vi "Process.vi"(8 "error in":errorcluster, 11 "SMO.Example":refnum<class "SMO.Example.lvclass">) -> (0 "error out":errorcluster, 3 "SMO.Example out":refnum<class "SMO.Example.lvclass">)   [LabVIEW 2013, in "SMO.Example.lvclass"]
doc: "---------------------------------------------------------------\nJKI State Machine Objects™\nhttp://jki.net/state-machine-objects/\nCopyright (C) 2005-2015, JKI <info@jki.net>\nALL RIGHTS RESERVED"
uses:
  SMO.Example.lvclass
  SMO/Typedefs/Parent Call--Enum.ctl
  SMO/SMO.lvclass
panel:
  # "For instructions on how to use the JKI State Machine Objects, examples and video tutorials, visit:\nhttp://jki.net/state-machine-objects/\n\nJKI State Machine Objects™\nhttp://jki.net/state-machine-objects/\nCopyright (C) 2005-2015, JKI <info@jki.net>\nALL RIGHTS RESERVED"
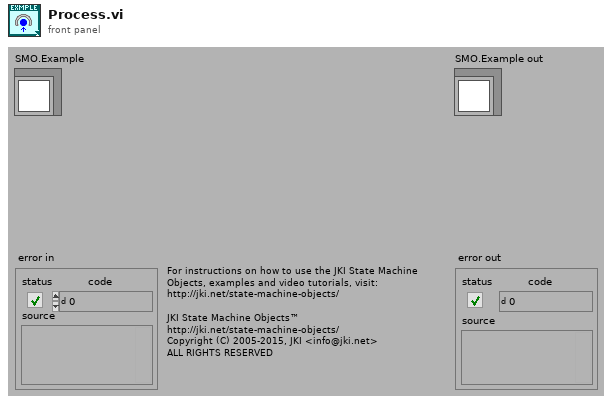
[diagram p1: front panel]
types:
  T1 = typedef "SMO.lvclass/Parent Call--Enum.ctl" = enum16{"Allows parent to run", "Does not request parent to run"}
  T2 = enum32{"invalid app kind", "Development System", "Run Time System", "Student Edition", "Embedded LabVIEW", "Evaluation", "Custom"}
  T3 = enum32{"Invalid", "Standard", "Closed", "Hidden", "Minimized", "Maximized"}
  T4 = enum32{"Bad", "Idle", "Run top level", "Running"}
  T5 = cluster{"Core":cluster{"Current VI Reference":refnum<vi>, "Close Panel on Exit?":bool, "error":errorcluster}, "Self Ref":refnum<class "SMO.Example.lvclass">, "Exec.State":enum32{"Bad", "Idle", "Run top level", "Running"}, "Your string data":string, "Pump State":bool, "Valve 1 State":bool, "Flow 1 Actual":dbl, "Flow 2 Actual":dbl, "Flow 1 Target":dbl, "Flow 2 Target":dbl}
  T6 = cluster{"Current VI Reference":refnum<vi>, "Close Panel on Exit?":bool, "error":errorcluster}
  T7 = typedef "SMO.lvclass/Protected Events.ctl" = cluster{"StopProcesses":refnum<user-event>, "AbortProcesses":refnum<user-event>}
  T8 = typedef "SMO.Example.lvclass/ProtectedEvents--Cluster.ctl" = cluster{"API_Template":refnum<user-event>, "PumpState":refnum<user-event>, "Valve State":refnum<user-event>}
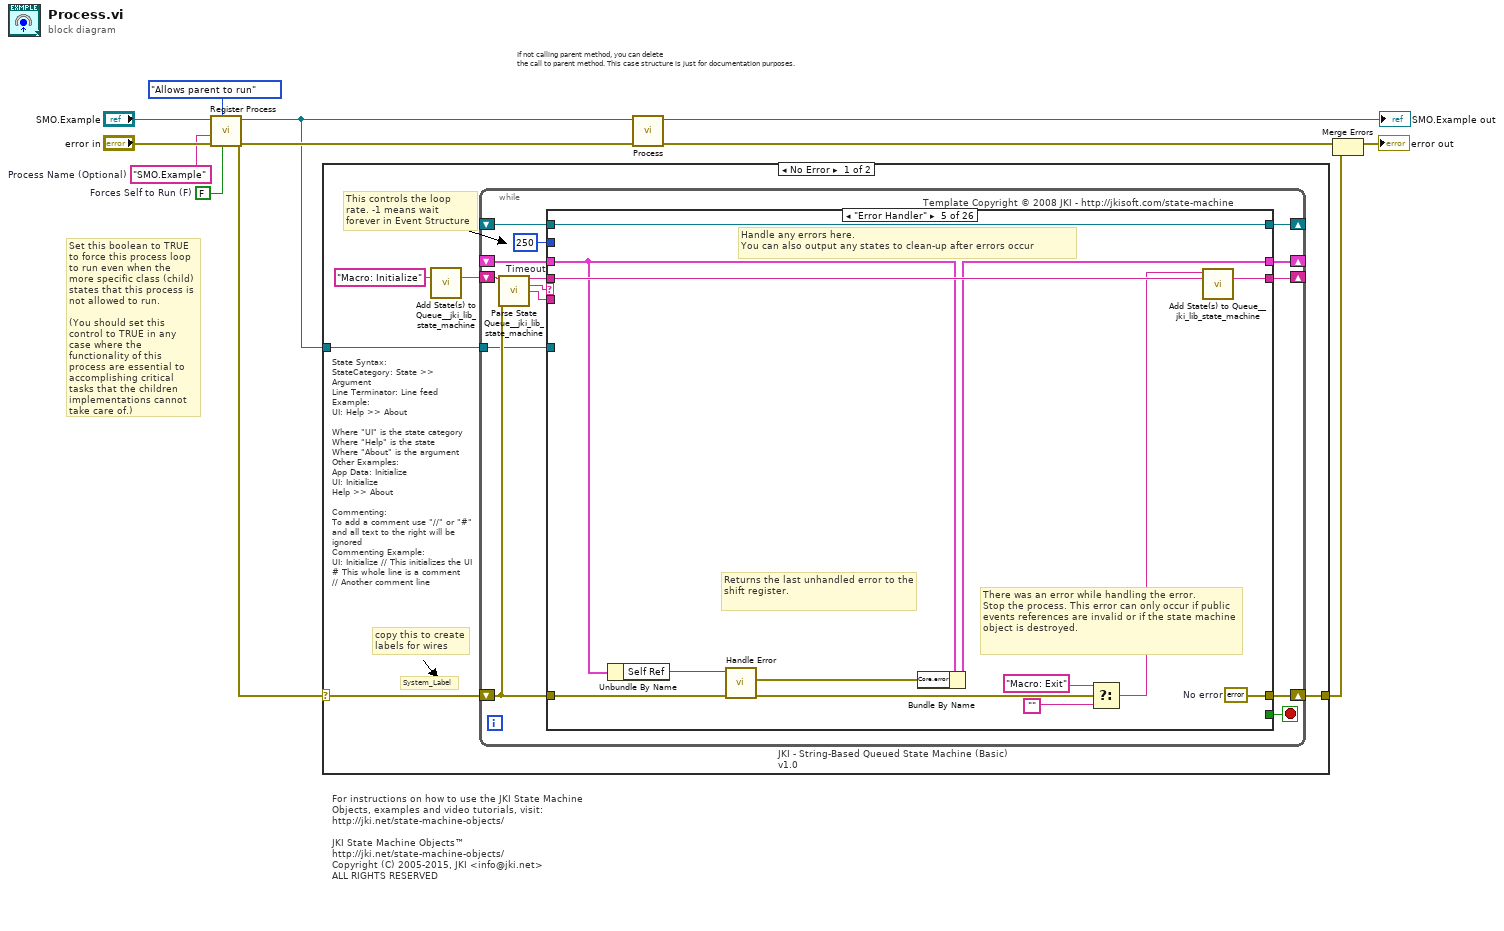
[diagram p0: block diagram]
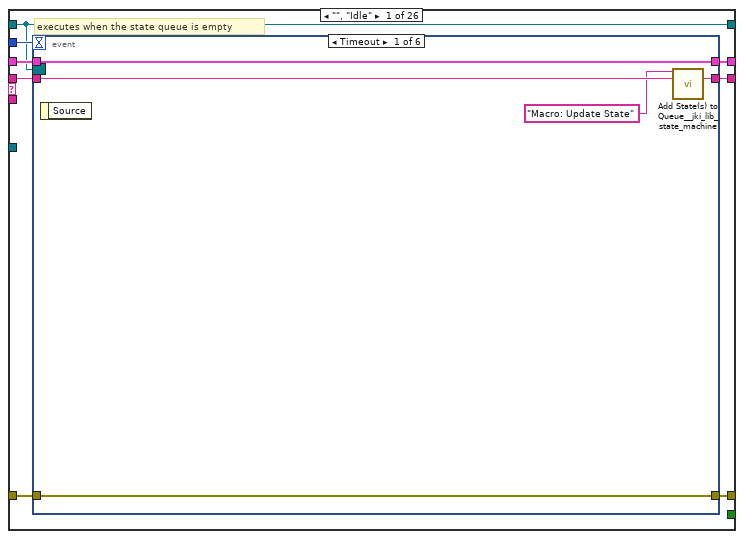
[diagram p2: hidden frame]
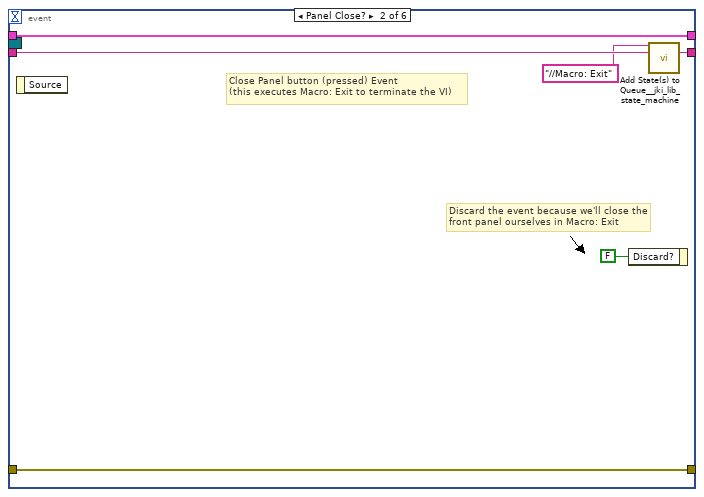
[diagram p3: hidden frame]
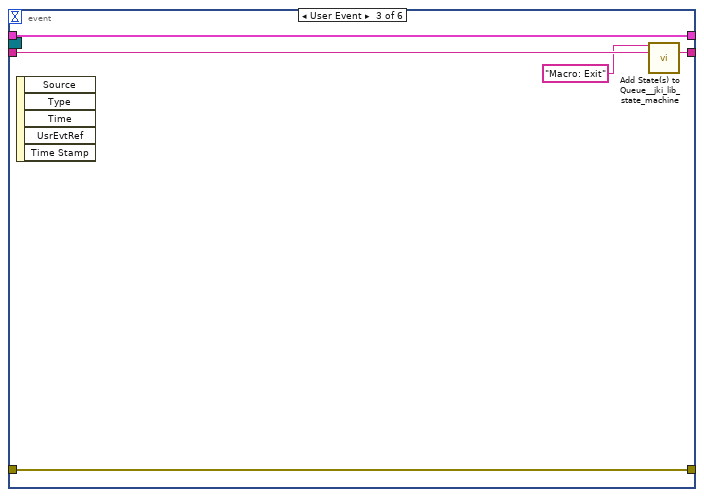
[diagram p4: hidden frame]
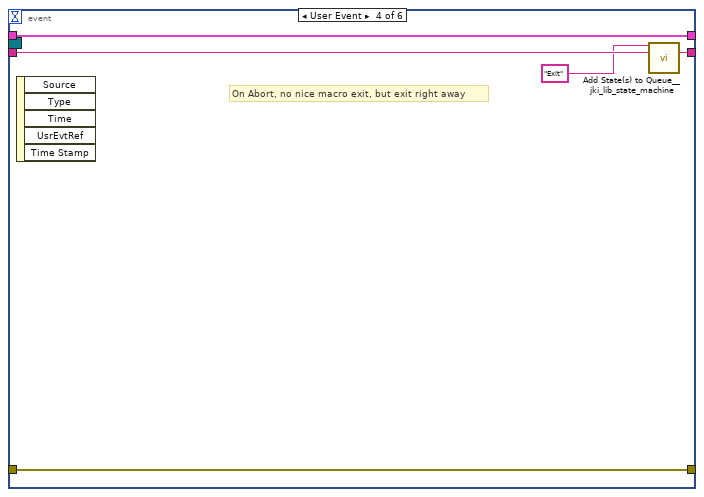
[diagram p5: hidden frame]
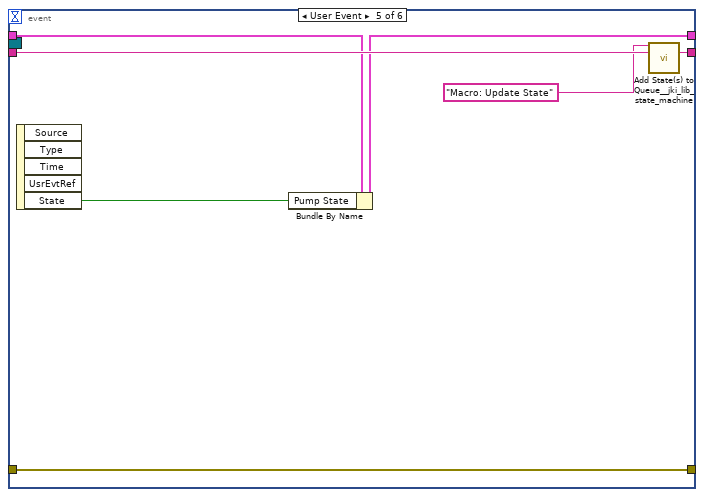
[diagram p6: hidden frame]
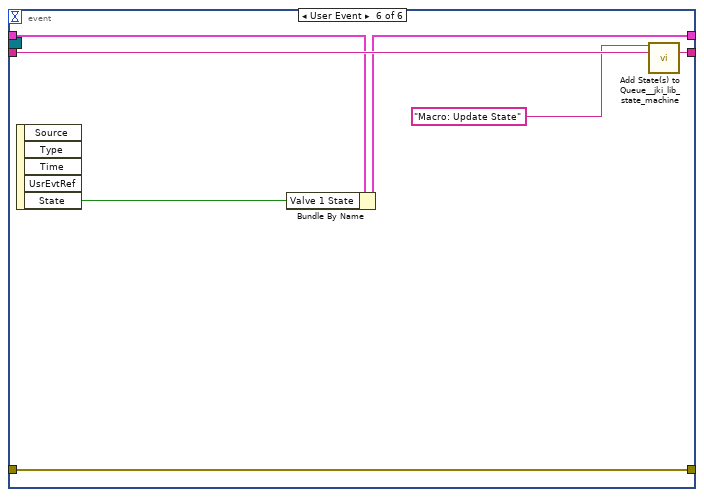
[diagram p7: hidden frame]
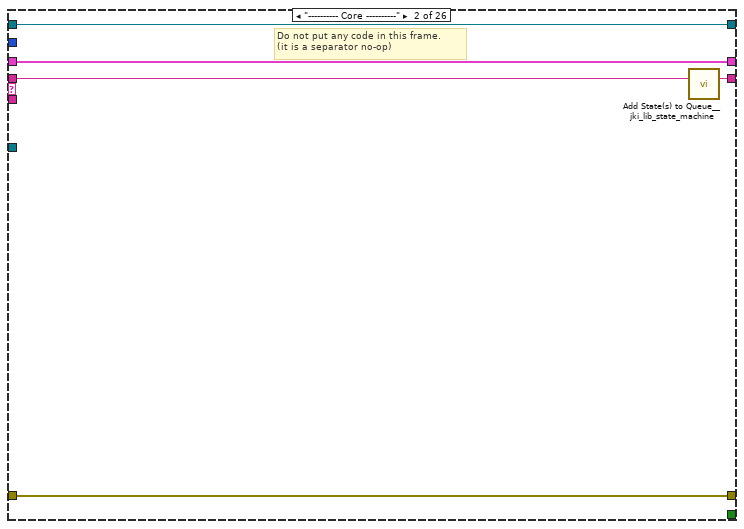
[diagram p8: hidden frame]
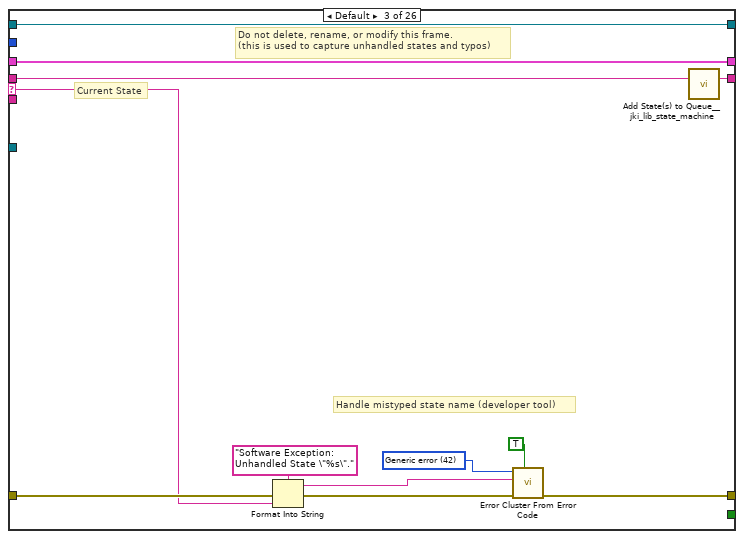
[diagram p9: hidden frame]
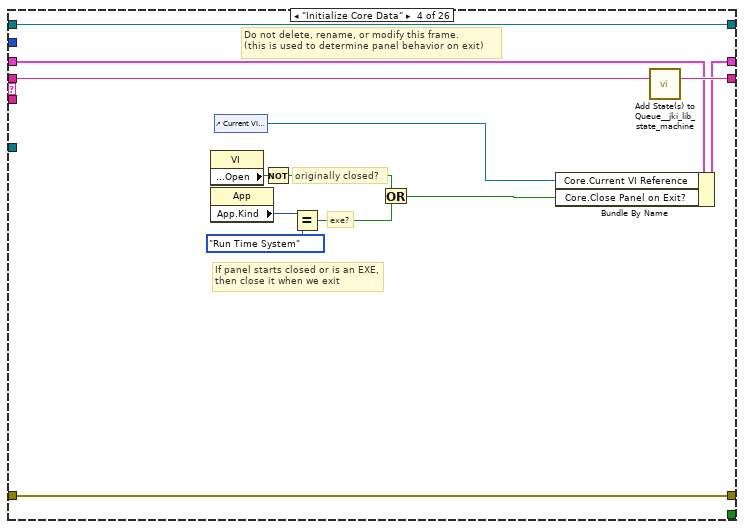
[diagram p10: hidden frame]
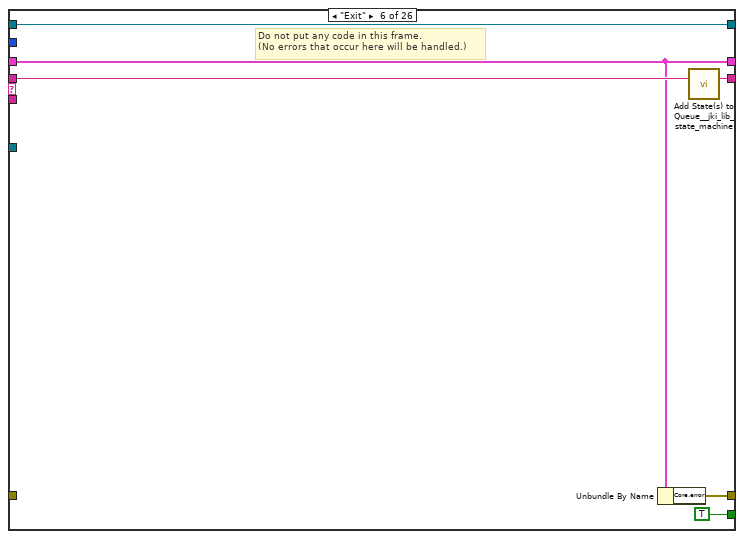
[diagram p11: hidden frame]
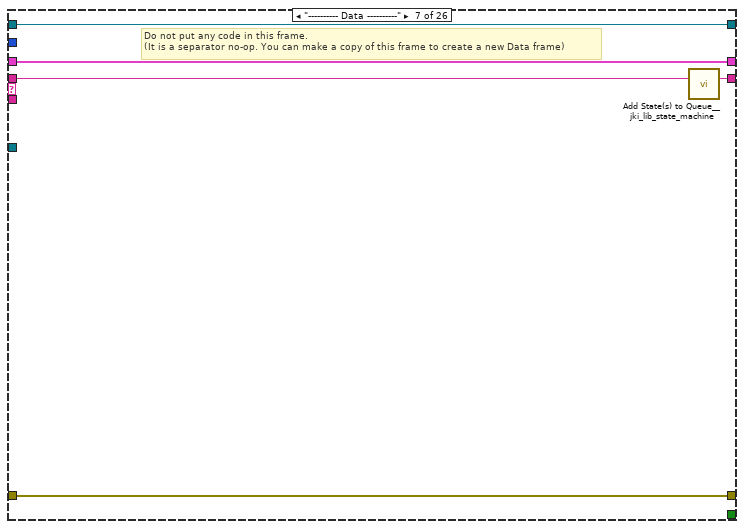
[diagram p12: hidden frame]
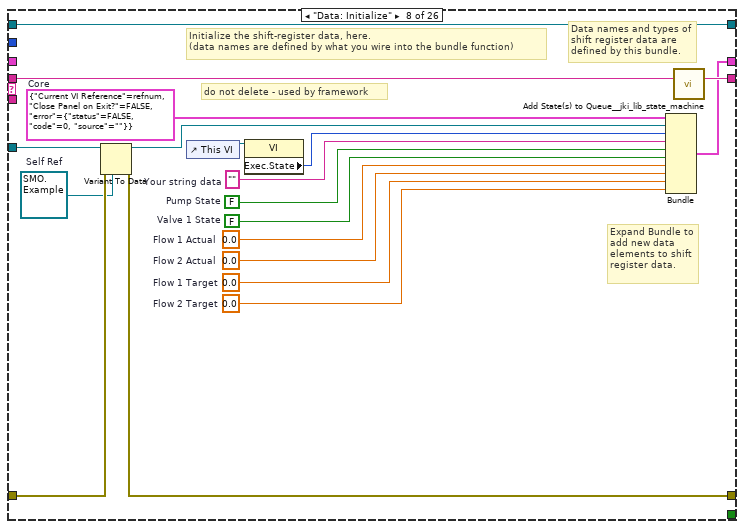
[diagram p13: hidden frame]
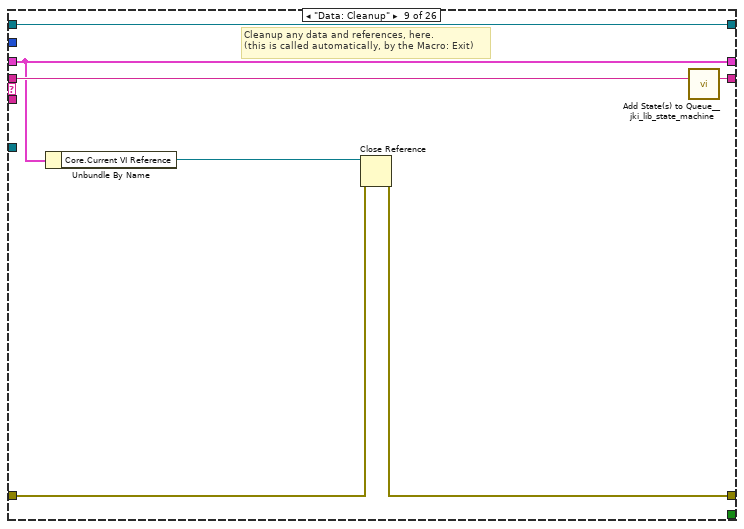
[diagram p14: hidden frame]
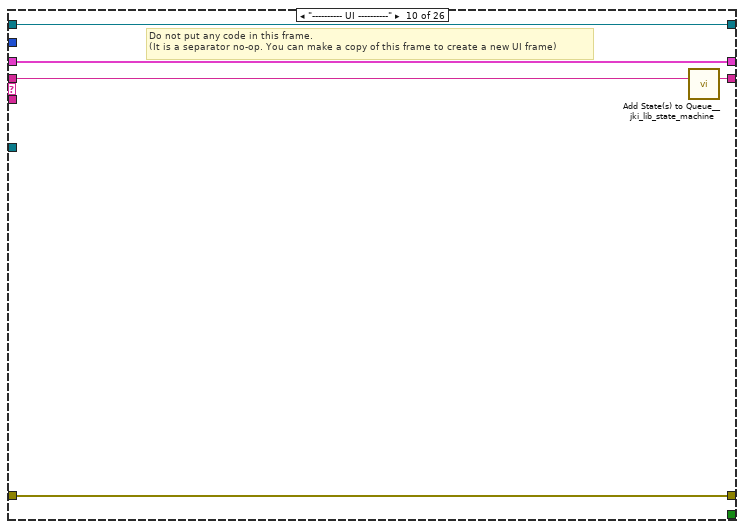
[diagram p15: hidden frame]
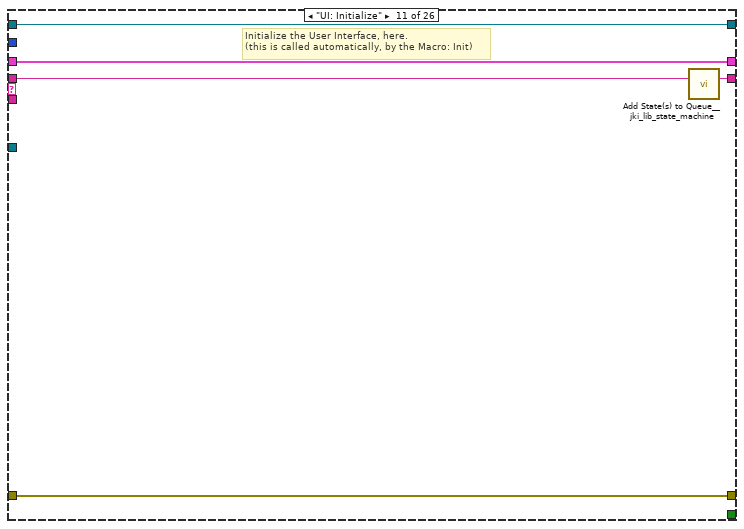
[diagram p16: hidden frame]
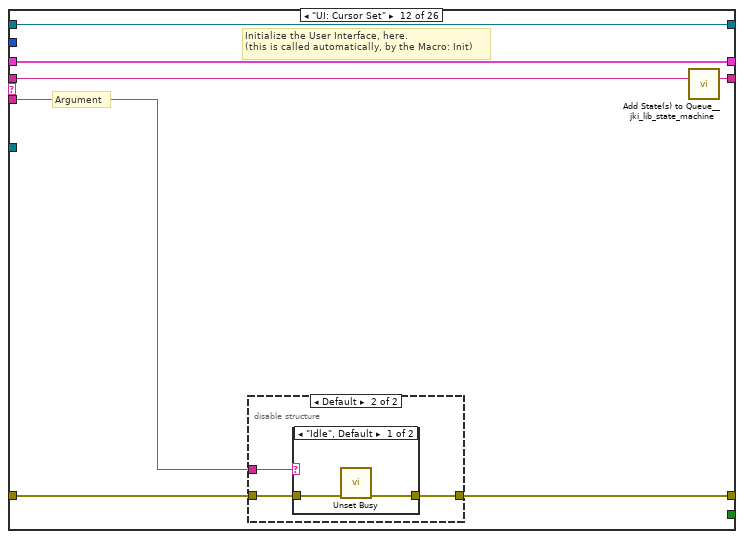
[diagram p17: hidden frame]
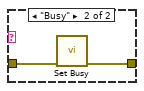
[diagram p19: hidden frame]
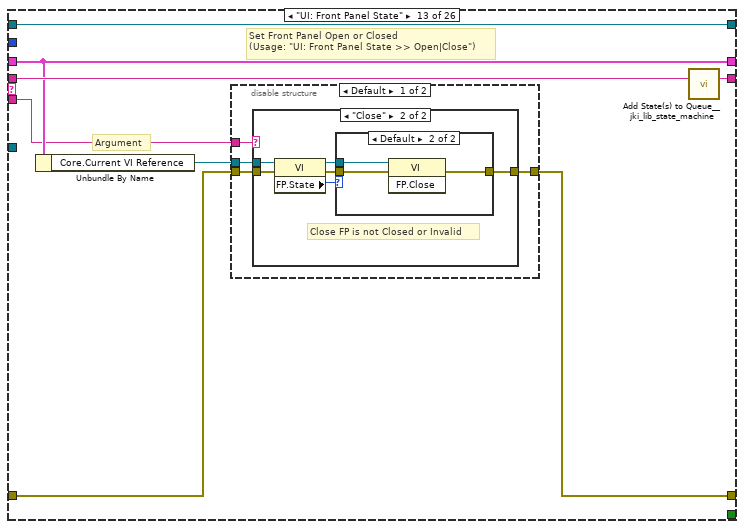
[diagram p20: hidden frame]
diagram:
  w1 = FALSE  # Forces Self to Run (F)
  w2 = "SMO.Example"  # Process Name (Optional)
  # "Set this boolean to TRUE to force this process loop to run even when the more specific class (child) states that this process is not allowed to run.\n\n(You should set this control to TRUE in any case where the functionality of this process are essential to accomplishing critical tasks that the children implementations cannot take care of.)"
  # "If not calling parent method, you can delete\nthe call to parent method. This case structure is just for documentation purposes."
  # "For instructions on how to use the JKI State Machine Objects, examples and video tutorials, visit:\nhttp://jki.net/state-machine-objects/\n\nJKI State Machine Objects™\nhttp://jki.net/state-machine-objects/\nCopyright (C) 2005-2015, JKI <info@jki.net>\nALL RIGHTS RESERVED"
  n1 = call "Register Process.vi"("Forces Self to Run (F)"=w1, "Parent Call"=Parent_Call--Enum."Allows parent to run", "error in (no error)"="error in", "Process Name (Optional)"=w2, "SMO"="SMO.Example") -> ("error out"=w8:errorcluster, "SMO out"=w7:refnum<class "SMO.Example.lvclass">)  [unwired: 5 in]
  n2 = case shown="No Error" w8 {
    selector: w8 -> [w13 w361]
    tunnel: w7 -> [w14 _]
    tunnel: [w12 w361] -> w4
    frame No Error {
      # "State Syntax:\nStateCategory: State >> Argument\nLine Terminator: Line feed\nExample:\nUI: Help >> About\n\nWhere \"UI\" is the state category\nWhere \"Help\" is the state\nWhere \"About\" is the argument\nOther Examples:\nApp Data: Initialize\nUI: Initialize\nHelp >> About\n\nCommenting:\nTo add a comment use \"//\" or \"#\" and all text to the right will be ignored\nCommenting Example:\nUI: Initialize // This initializes the UI\n# This whole line is a comment\n// Another comment line"
      # "copy this to create labels for wires"
      # "This controls the loop rate. -1 means wait forever in Event Structure"
      # "System_Label"
      n3 = call <vilib>:"Add State(s) to Queue__jki_lib_state_machine.vi"("State(s) in (\"\")"="Macro: Initialize") -> ("States Out"=w16:string)  [unwired: 14 in]
      n4 = while "JKI - String-Based Queued State Machine (Basic) v1.0" {
        shift-right: [w23] -> _
        shift-left: _ -> [w22]
        shift-right: [w26] -> w12
        shift-left: w13 -> [w20]
        shift-right: [w25] -> _
        shift-left: w16 -> [w27]
        tunnel: w14 -> [w19]
        shift-right: [w18] -> _
        shift-left: _ -> [w17]
        stop <- w24 stop-if-true
        w21 = 250  # Timeout
        # "Template Copyright © 2008 JKI - http://jkisoft.com/state-machine"
        n5 = call <vilib>:"Parse State Queue__jki_lib_state_machine.vi"("State Queue"=w27, "Error In (no error)"=w20) -> ("Remaining States"=w29:string, "Current State"=w30:string, "Arguments"=w28:string)  [unwired: 11 in]
        n6 = case shown="\"Error Handler\"" w30 {
          selector: w30 -> [_ _ w80 _ _ _ _ _ _ _ _ _ _ _ _ _ _ _ _ _ _ _ _ _ _ _]
          tunnel: w29 -> [w38 w78 w84 w103 w116 w122 w127 w146 w153 w158 w163 w170 w186 w218 w224 w238 w256 w261 w272 w282 w294 w300 w305 w315 w351 w360]
          tunnel: w28 -> [_ _ _ _ _ _ _ _ _ _ _ w164 w182 _ _ _ _ _ _ _ _ _ _ _ _ _]
          tunnel: w22 -> [w36 w75 w82 w94 w107 w118 w124 _ w148 w155 w161 w168 w184 w215 w221 w234 w243 w258 w268 w279 w292 w298 w303 w309 w347 w357]
          tunnel: [w35 w76 w86 w100 w104 w117 w125 w141 w149 w156 w160 w165 w179 w216 w222 w236 w254 w259 w269 w280 w291 w295 w301 w310 w348 w354] -> w26
          tunnel: w20 -> [w34 w76 w85 w100 w108 _ w125 w142 w150 w156 w160 w166 w180 w216 w222 w236 w254 w259 w265 w280 w286 w296 w301 w310 w348 w355]
          tunnel: [w37 w77 w83 w102 w115 w121 w126 w145 w152 w157 w162 w169 w185 w217 w223 w237 w255 w260 w271 w281 w293 w299 w304 w314 w350 w359] -> w25
          tunnel: [_ _ _ _ _ TRUE _ _ _ _ _ _ _ _ _ _ _ _ _ _ _ _ _ _ _ _] -> w24
          tunnel: [w33 w75 w82 w101 w106 w118 w124 w144 w148 w155 w161 w168 w184 w215 w221 w234 w243 w258 w268 w279 w292 w298 w303 w308 w346 w357] -> w23
          tunnel: w21 -> [w32 _ _ _ _ _ _ _ _ _ _ _ _ _ _ _ _ _ _ _ _ _ _ _ _ _]
          tunnel: w19 -> [_ _ _ _ _ _ _ w139 _ _ _ _ _ _ _ _ _ _ _ _ _ _ _ _ _ _]
          tunnel: [w31 w74 w79 w91 w114 w119 w123 w137 w147 w154 w159 w167 w183 w214 w220 w235 w248 w257 w270 w278 w284 w297 w302 w313 w349 w358] -> w18
          tunnel: w17 -> [w31 w74 w79 w91 w114 w119 w123 w137 w147 w154 w159 w167 w183 w214 w220 w235 w248 w257 w270 w278 _ w297 w302 w313 w349 w358]
          frame "", "Idle" {
            # "executes when the state queue is empty"
            n7 = event shown="[0] Timeout" {
              selector: w31 -> [_ _ _ _ _ _]
              dyn-events: _ -> [_ _ _ _ _ _]
              timeout: w32 -> [_ _ _ _ _ _]
              tunnel: w38 -> [w43 w49 w54 w59 w66 w73]
              tunnel: [w42 w48 w53 w58 w65 w72] -> w37
              tunnel: w36 -> [w40 w46 w51 w56 w63 w70]
              tunnel: [w41 w47 w52 w57 w64 w71] -> w35
              tunnel: w34 -> [w41 w47 w52 w57 w64 w71]
              tunnel: [w40 w46 w51 w56 w62 w69] -> w33
              event Timeout {
                n8 = event-data() -> ()  [unwired: 1 in, 1 out]
                n9 = call <vilib>:"Add State(s) to Queue__jki_lib_state_machine.vi"("State(s) in Front (\"\")"="Macro: Update State", "State(s) in (\"\")"=w43) -> ("States Out"=w42:string)  [unwired: 13 in]
              }
              event Panel Close? {
                # "Discard the event because we'll close the front panel ourselves in Macro: Exit"
                # "Close Panel button (pressed) Event\n(this executes Macro: Exit to terminate the VI)"
                n10 = event-data() -> ()  [unwired: 1 in, 1 out]
                n11 = event-data("Discard?"=FALSE) -> ()  [unwired: 1 in, 1 out]
                n12 = call <vilib>:"Add State(s) to Queue__jki_lib_state_machine.vi"("State(s) in Front (\"\")"="//Macro: Exit", "State(s) in (\"\")"=w49) -> ("States Out"=w48:string)  [unwired: 13 in]
              }
              event User Event {
                n13 = event-data() -> ()  [unwired: 1 in, 5 out]
                n14 = call <vilib>:"Add State(s) to Queue__jki_lib_state_machine.vi"("State(s) in Front (\"\")"="Macro: Exit", "State(s) in (\"\")"=w54) -> ("States Out"=w53:string)  [unwired: 13 in]
              }
              event User Event {
                # "On Abort, no nice macro exit, but exit right away"
                n15 = event-data() -> ()  [unwired: 1 in, 5 out]
                n16 = call <vilib>:"Add State(s) to Queue__jki_lib_state_machine.vi"("State(s) in Front (\"\")"="Exit", "State(s) in (\"\")"=w59) -> ("States Out"=w58:string)  [unwired: 13 in]
              }
              event User Event {
                n17 = event-data() -> ("State"=w60:bool)  [unwired: 1 in, 4 out]
                n18 = Bundle By Name(cluster=w63, "Pump State"=w60) -> (w62:T5)
                n19 = call <vilib>:"Add State(s) to Queue__jki_lib_state_machine.vi"("State(s) in Front (\"\")"="Macro: Update State", "State(s) in (\"\")"=w66) -> ("States Out"=w65:string)  [unwired: 13 in]
              }
              event User Event {
                n20 = event-data() -> ("State"=w67:bool)  [unwired: 1 in, 4 out]
                n21 = Bundle By Name(cluster=w70, "Valve 1 State"=w67) -> (w69:T5)
                n22 = call <vilib>:"Add State(s) to Queue__jki_lib_state_machine.vi"("State(s) in Front (\"\")"="Macro: Update State", "State(s) in (\"\")"=w73) -> ("States Out"=w72:string)  [unwired: 13 in]
              }
            }
          }
          frame "---------- Core ----------" {
            # "Do not put any code in this frame.\n(it is a separator no-op)"
            n23 = call <vilib>:"Add State(s) to Queue__jki_lib_state_machine.vi"("State(s) in (\"\")"=w78) -> ("States Out"=w77:string)  [unwired: 14 in]
          }
          frame Default {
            w89 = 42 items=["No error", "Argument error", "Memory is full", "Out of zone", "End of file", "File already open", "Generic file I/O error", "File not found", "File permission error", "Disk is full", "Duplicate path", "Too many files open", "System feature not enabled", "Resource file not found", "Cannot add resource", "Resource not found", "Image not found", "Image memory error", "Pen does not exist", "Config type invalid", "Config token not found", "Config parse error", "Config memory error", "Bad external code format", "Bad external code offset", "External code not present", "Null window", "Destroy window error", "Null menu", "Print aborted", "Bad print record", "Print driver error", "Windows error during printing", "Memory error during printing", "Print dialog error", "Generic print error", "Invalid device refnum", "Device not found", "Device parameter error", "Device unit error", "Cannot open device", "Device call aborted", "Generic error", "Cancelled by user", "Object ID too low", "Object ID too high", "Object not in heap", "Unknown heap", "Unknown object (invalid DefProc)", "Unknown object (DefProc not in table)", "Message out of range", "Invalid (null) method", "Unknown message", "Manager call not supported", "Bad address", "Network operation in progress", "Network operation timed out", "Connection is busy", "Network attribute not supported", "Network error", "Address in use", "System out of memory", "Connection aborted", "Connection refused", "Not connected", "Already connected", "Connection closed", "Initialization error (interapplication manager)", "Bad occurrence", "Wait on unbound occurrence handler", "Occurrence queue overflow", "Datalog type conflict", "Unused", "Unrecognized type (interapplication manager)", "Memory corrupt", "Failed to make temporary DLL", "Old CIN version", "Drag socket not found", "Failed to load drop-object", "Failed to register OLE object", "Failed to release OLE object", "Format specifier type mismatch", "Unknown format specifier", "Too few format specifiers", "Too many format specifiers", "Scan failed", "Newer CIN version", "Error converting to variant", "Runtime menu error", "Password tampered", "Variant attribute not found", "Incompatible variant data type", "Event data is not available", "Event Store is not present", "Occurrence is not found", "Event Queue is not created", "Event info is not available", "Refnum passed is NULL", "Error retrieving Class GUID", "Error retrieving CoClass GUID", "Error retrieving TypeLib GUID.", "Bad built application magic bytes.", "Specific driver is different from the specific driver associated with the Logical Name.", "There is no session opened to the class driver.", "Max Error", "MAX - Error with config objects", "MAX - Error loading configuration", "MAX - Group not supported"]
            # "Current State"
            # "Do not delete, rename, or modify this frame.\n(this is used to capture unhandled states and typos)"
            # "Handle mistyped state name (developer tool)"
            n24 = Format Into String(format string="Software Exception: Unhandled State \"%s\"." ("message"), error in=w85, w80) -> (resulting string=w88:string, error out=w87:errorcluster)  [unwired: 1 in]
            n25 = call <vilib>:"Error Cluster From Error Code.vi"("show call chain? (False)"=TRUE, "error in (no error)"=w87, "error message (\"\")"=w88, "error code (0)"=w89) -> ("error out"=w86:errorcluster)  [unwired: 5 in]
            n26 = call <vilib>:"Add State(s) to Queue__jki_lib_state_machine.vi"("State(s) in (\"\")"=w84) -> ("States Out"=w83:string)  [unwired: 14 in]
          }
          frame "Initialize Core Data" {
            # "Do not delete, rename, or modify this frame.\n(this is used to determine panel behavior on exit)"
            # "originally closed?"
            # "exe?"
            # "If panel starts closed or is an EXE, then close it when we exit"
            n27 = property class="VI"() -> ("Front Panel.Open"=w99:bool)  [unwired: 2 in, 2 out]
            n28 = property class="App"() -> ("App.Kind"=w98:T2)  [unwired: 2 in, 2 out]
            n29 = control-ref of="Current VI Reference"() -> (w92:refnum<vi>)
            n30 = Not(x=w99) -> (.not. x?=w96:bool)
            n31 = Equal?(x=w98, y=T2."Run Time System" ("Application:Kind")) -> (x = y?=w95:bool)
            n32 = Or(x=w96, y=w95) -> (x .or. y?=w93:bool)
            n33 = Bundle By Name(cluster=w94, "Core.Current VI Reference"=w92, "Core.Close Panel on Exit?"=w93) -> (w101:T5)
            n34 = call <vilib>:"Add State(s) to Queue__jki_lib_state_machine.vi"("State(s) in (\"\")"=w103) -> ("States Out"=w102:string)  [unwired: 14 in]
          }
          frame "Error Handler" {
            w104 = errorcluster {"status"=FALSE, "code"=0, "source"=""}  # No error
            # "Returns the last unhandled error to the shift register."
            # "There was an error while handling the error.\nStop the process. This error can only occur if public events references are invalid or if the state machine object is destroyed."
            # "Handle any errors here.\nYou can also output any states to clean-up after errors occur"
            n35 = Unbundle By Name(w107) -> ("Self Ref"=w109:refnum<class "SMO.Example.lvclass">)
            n36 = call-dynamic "Handle Error.vi"("error in"=w108, "SMO"=w109) -> ("handling error"=w111:errorcluster, "Unhandled error"=w110:errorcluster)  [unwired: 7 in, 1 out]
            n37 = Bundle By Name(cluster=w107, "Core.error"=w110) -> (w106:T5)
            n38 = Select(t="Macro: Exit", s=w111, f="") -> (s? t:f=w105:string)
            n39 = call <vilib>:"Add State(s) to Queue__jki_lib_state_machine.vi"("State(s) in Front (\"\")"=w105, "State(s) in (\"\")"=w116) -> ("States Out"=w115:string)  [unwired: 13 in]
          }
          frame "Exit" {
            # "Do not put any code in this frame.\n(No errors that occur here will be handled.)"
            n40 = Unbundle By Name(w118) -> ("Core.error"=w117:errorcluster)
            n41 = call <vilib>:"Add State(s) to Queue__jki_lib_state_machine.vi"("State(s) in (\"\")"=w122) -> ("States Out"=w121:string)  [unwired: 14 in]
          }
          frame "---------- Data ----------" {
            # "Do not put any code in this frame.\n(It is a separator no-op. You can make a copy of this frame to create a new Data frame)"
            n42 = call <vilib>:"Add State(s) to Queue__jki_lib_state_machine.vi"("State(s) in (\"\")"=w127) -> ("States Out"=w126:string)  [unwired: 14 in]
          }
          frame "Data: Initialize" {
            w128 = T6 {"Current VI Reference"=refnum, "Close Panel on Exit?"=FALSE, "error"={"status"=FALSE, "code"=0, "source"=""}}  # Core
            w129 = 0.0  # Flow 2 Target
            w130 = 0.0  # Flow 1 Target
            w131 = 0.0  # Flow 2 Actual
            w132 = 0.0  # Flow 1 Actual
            w133 = FALSE  # Valve 1 State
            w134 = FALSE  # Pump State
            w140 = refnum<class "SMO.Example.lvclass"> refnum  # Self Ref
            w143 = ""  # Your string data
            # "do not delete - used by framework"
            # "Expand Bundle to add new data elements to shift register data."
            # "Data names and types of shift register data are defined by this bundle."
            # "Initialize the shift-register data, here.\n(data names are defined by what you wire into the bundle function)"
            n43 = Variant To Data(error in=w142, type=w140, Variant=w139) -> (data=w138:refnum<class "SMO.Example.lvclass">, error out=w141:errorcluster)
            n44 = control-ref of="This VI"() -> (w135:refnum<vi>)
            n45 = property class="VI"(reference=w135) -> ("Exec.State"=w136:T4)  [unwired: 1 in, 2 out]
            n46 = Bundle("Core"=w128, "Self Ref"=w138, "Exec.State"=w136, "Your string data"=w143, "Pump State"=w134, "Valve 1 State"=w133, "Flow 1 Actual"=w132, "Flow 2 Actual"=w131, "Flow 1 Target"=w130, "Flow 2 Target"=w129) -> (w144:T5)  [unwired: 1 in]
            n47 = call <vilib>:"Add State(s) to Queue__jki_lib_state_machine.vi"("State(s) in (\"\")"=w146) -> ("States Out"=w145:string)  [unwired: 14 in]
          }
          frame "Data: Cleanup" {
            # "Cleanup any data and references, here.\n(this is called automatically, by the Macro: Exit)"
            n48 = Unbundle By Name(w148) -> ("Core.Current VI Reference"=w151:refnum<vi>)
            n49 = Close Reference(reference=w151, error in (no error)=w150) -> (error out=w149:errorcluster)
            n50 = call <vilib>:"Add State(s) to Queue__jki_lib_state_machine.vi"("State(s) in (\"\")"=w153) -> ("States Out"=w152:string)  [unwired: 14 in]
          }
          frame "---------- UI ----------" {
            # "Do not put any code in this frame.\n(It is a separator no-op. You can make a copy of this frame to create a new UI frame)"
            n51 = call <vilib>:"Add State(s) to Queue__jki_lib_state_machine.vi"("State(s) in (\"\")"=w158) -> ("States Out"=w157:string)  [unwired: 14 in]
          }
          frame "UI: Initialize" {
            # "Initialize the User Interface, here.\n(this is called automatically, by the Macro: Init)"
            n52 = call <vilib>:"Add State(s) to Queue__jki_lib_state_machine.vi"("State(s) in (\"\")"=w163) -> ("States Out"=w162:string)  [unwired: 14 in]
          }
          frame "UI: Cursor Set" {
            # "Argument"
            # "Initialize the User Interface, here.\n(this is called automatically, by the Macro: Init)"
            n53 = disable-structure shown="Default" {
              disable-tunnel: w166 -> [w171 w174]
              disable-tunnel: [w171 w173] -> w165
              disable-tunnel: w164 -> [_ w172]
              frame condition #0 {
              }
              frame condition #1 (active) {
                n54 = case shown="\"Idle\", Default" w172 {
                  tunnel: w174 -> [w176 w178]
                  tunnel: [w175 w177] -> w173
                  frame "Idle", Default {
                    n55 = call <vilib>:"Unset Busy.vi"("error in (no error)"=w176) -> ("error out"=w175:errorcluster)  [unwired: 10 in]
                  }
                  frame "Busy" {
                    n56 = call <vilib>:"Set Busy.vi"("error in (no error)"=w178) -> ("error out"=w177:errorcluster)  [unwired: 9 in, 1 out]
                  }
                }
              }
            }
            n57 = call <vilib>:"Add State(s) to Queue__jki_lib_state_machine.vi"("State(s) in (\"\")"=w170) -> ("States Out"=w169:string)  [unwired: 14 in]
          }
          frame "UI: Front Panel State" {
            # "Argument"
            # "Set Front Panel Open or Closed\n(Usage: \"UI: Front Panel State >> Open|Close\")"
            n58 = Unbundle By Name(w184) -> ("Core.Current VI Reference"=w181:refnum<vi>)
            n59 = disable-structure shown="Default" {
              disable-tunnel: w180 -> [w190 w213]
              disable-tunnel: [w189 w213] -> w179
              disable-tunnel: w181 -> [w188 _]
              disable-tunnel: w182 -> [w187 _]
              frame condition #0 (active) {
                n60 = case shown="\"Close\"" w187 {
                  tunnel: w190 -> [w194 w207]
                  tunnel: [w196 w208] -> w189
                  tunnel: w188 -> [w195 w205]
                  frame "Open", Default {
                    # "Open FP if not open or invalid"
                    n61 = property class="VI"(reference=w195, error in=w194) -> (reference out=w192:refnum<vi>, error out=w193:errorcluster, "FP.State"=w191:T3)
                    n62 = case shown="Default" w191 {
                      tunnel: [w199 w202] -> w196
                      tunnel: w193 -> [w198 w202]
                      tunnel: w192 -> [w197 _]
                      frame Default {
                        n63 = invoke class="VI" method="FP.Open"(reference=w197, error in=w198, "Activate"=TRUE, "State"=T3."Standard") -> (error out=w199:errorcluster)  [unwired: 1 in, 4 out]
                      }
                      frame "Invalid", "Standard" {
                      }
                    }
                  }
                  frame "Close" {
                    # "Close FP is not Closed or Invalid"
                    n64 = property class="VI"(reference=w205, error in=w207) -> (reference out=w204:refnum<vi>, error out=w206:errorcluster, "FP.State"=w203:T3)
                    n65 = case shown="Default" w203 {
                      tunnel: [w209 w212] -> w208
                      tunnel: w206 -> [w209 w211]
                      tunnel: w204 -> [_ w210]
                      frame "Invalid", "Closed" {
                      }
                      frame Default {
                        n66 = invoke class="VI" method="FP.Close"(reference=w210, error in=w211) -> (error out=w212:errorcluster)  [unwired: 1 in, 2 out]
                      }
                    }
                  }
                }
              }
              frame condition #1 {
              }
            }
            n67 = call <vilib>:"Add State(s) to Queue__jki_lib_state_machine.vi"("State(s) in (\"\")"=w186) -> ("States Out"=w185:string)  [unwired: 14 in]
          }
          frame "---------- Macro ----------" {
            # "Do not put any code in this frame.\n(It is a separator no-op. You can make a copy of this frame to create a new Macro frame)"
            n68 = call <vilib>:"Add State(s) to Queue__jki_lib_state_machine.vi"("State(s) in (\"\")"=w218) -> ("States Out"=w217:string)  [unwired: 14 in]
          }
          frame "Macro: Update State" {
            n69 = call <vilib>:"Add State(s) to Queue__jki_lib_state_machine.vi"("State(s) in Front (\"\")"="API: Determine Flow Targets\nAPI: Determine Actual Flow\nAPI: Update State", "State(s) in (\"\")"=w224) -> ("States Out"=w223:string)  [unwired: 13 in]
          }
          frame "Macro: Initialize" {
            w229 = "//UI: Initialize\n//UI: Front Panel State >> Open"  # //UI: Initialize //UI: Front Panel State >> Open
            w225 = "Process: Sync"
            # "Initialization Macro\n(This is called once, when the VI starts)"
            n70 = control-ref of="This VI"() -> (w227:refnum<vi>)
            n71 = property class="VI"(reference=w227) -> ("Exec.State"=w226:T4)  [unwired: 1 in, 2 out]
            n72 = Equal?(x=w226, y=T4."Run top level") -> (x = y?=w232:bool)
            n73 = Select(t=w225, s=w232, f="") -> ()  [unwired: 1 out]
            n74 = call <vilib>:"Add State(s) to Queue__jki_lib_state_machine.vi"("State(s) in Front (\"\")"="Data: Initialize\nInitialize Core Data\nEvents: Register", "State(s) in (\"\")"=w225, "State(s) at Back (\"\")"=w229) -> ("States Out"=w228:string)  [unwired: 12 in]
            n75 = call <vilib>:"Add State(s) to Queue__jki_lib_state_machine.vi"("State(s) in Front (\"\")"=w228, "State(s) in (\"\")"=w238) -> ("States Out"=w237:string)  [unwired: 13 in]
          }
          frame "Macro: Exit" {
            w239 = "Process: Sync"
            # "Exit Macro\n(This is called once, when the VI exits)"
            n76 = Unbundle By Name(w243) -> ("Core.Close Panel on Exit?"=w253:bool)
            n77 = Unbundle By Name(w243) -> ("Exec.State"=w247:T4)
            n78 = Equal?(x=w247, y=T4."Run top level") -> (x = y?=w245:bool)
            n79 = Select(t=w239, s=w245, f="") -> ()  [unwired: 1 out]
            n80 = Select(t="UI: Front Panel State >> Close", s=w253, f="") -> (s? t:f=w250:string)
            n81 = call <vilib>:"Add State(s) to Queue__jki_lib_state_machine.vi"("State(s) in Front (\"\")"="Data: Cleanup\nEvents: Unregister", "State(s) in (\"\")"=w239, "State(s) at Back (\"\")"="Exit") -> ("States Out"=w240:string)  [unwired: 12 in]
            n82 = call <vilib>:"Add State(s) to Queue__jki_lib_state_machine.vi"("State(s) in (\"\")"=w250, "State(s) at Back (\"\")"=w240) -> ("States Out"=w249:string)  [unwired: 13 in]
            n83 = call <vilib>:"Add State(s) to Queue__jki_lib_state_machine.vi"("State(s) in Front (\"\")"=w249, "State(s) in (\"\")"=w256) -> ("States Out"=w255:string)  [unwired: 13 in]
          }
          frame "---------- Process ----------" {
            # "Template Separator\n(You can make a copy of, or modify, this frame)"
            n84 = call <vilib>:"Add State(s) to Queue__jki_lib_state_machine.vi"("State(s) in (\"\")"=w261) -> ("States Out"=w260:string)  [unwired: 14 in]
          }
          frame "Process: Sync" {
            # "Template Separator\n(You can make a copy of, or modify, this frame)"
            n85 = Unbundle By Name(w268) -> ("Self Ref"=w267:refnum<class "SMO.Example.lvclass">)
            n86 = call "isProcessAllowedRun.vi"("error in (no error)"=w265, "SMO in"=w267) -> ("error out"=w264:errorcluster, "Run Allowed"=w263:bool, "SMO out"=w266:refnum<class "SMO.Example.lvclass">)  [unwired: 7 in]
            n87 = case shown="True" w263 {
              tunnel: [w274 w277] -> w269
              tunnel: w266 -> [_ w276]
              tunnel: w264 -> [w274 w275]
              tunnel: ["Macro: Exit" _] -> w262
              frame False {
              }
              frame True {
                n88 = call "WaitOnProcessSync.vi"("error in (no error)"=w275, "SMO"=w276) -> ("error out"=w277:errorcluster)  [unwired: 8 in, 1 out]
              }
            }
            n89 = call <vilib>:"Add State(s) to Queue__jki_lib_state_machine.vi"("State(s) in Front (\"\")"=w262, "State(s) in (\"\")"=w272) -> ("States Out"=w271:string)  [unwired: 13 in]
          }
          frame "---------- Events ----------" {
            # "Template Separator\n(You can make a copy of, or modify, this frame)"
            n90 = call <vilib>:"Add State(s) to Queue__jki_lib_state_machine.vi"("State(s) in (\"\")"=w282) -> ("States Out"=w281:string)  [unwired: 14 in]
          }
          frame "Events: Register" {
            # "Self Public Events"
            # "Base Class Protected Events"
            # "Your code here.\n(You can make a copy of, or modify, this frame)"
            n91 = Unbundle By Name(w292) -> ("Self Ref"=w289:refnum<class "SMO.Example.lvclass">)
            n92 = call "GetProtectedEvents.vi"("error in (no error)"=w286, "SMO"=w289) -> ("error out"=w285:errorcluster, "SMO Protected Events"=w288:T7, "SMO out"=w287:refnum<class "SMO.Example.lvclass">)  [unwired: 7 in]
            n93 = call "SMO.Example.GetProtectedEvents.vi"("error in (no error)"=w285, "SMO.Example"=w287) -> ("error out"=w290:errorcluster, "Protected Events"=w283:T8)  [unwired: 7 in, 1 out]
            n94 = register-events(error in=w290, w288, w283) -> (reference out=w284:refnum<event-registration>, error out=w291:errorcluster)  [unwired: 1 in]
            n95 = call <vilib>:"Add State(s) to Queue__jki_lib_state_machine.vi"("State(s) in (\"\")"=w294) -> ("States Out"=w293:string)  [unwired: 14 in]
          }
          frame "Events: Unregister" {
            # "Your code here.\n(You can make a copy of, or modify, this frame)"
            n96 = Unregister For Events(event registration refnum=w297, error in=w296) -> (error out=w295:errorcluster)
            n97 = call <vilib>:"Add State(s) to Queue__jki_lib_state_machine.vi"("State(s) in (\"\")"=w300) -> ("States Out"=w299:string)  [unwired: 14 in]
          }
          frame "---------- API ----------" {
            n98 = call <vilib>:"Add State(s) to Queue__jki_lib_state_machine.vi"("State(s) in (\"\")"=w305) -> ("States Out"=w304:string)  [unwired: 14 in]
          }
          frame "API: Determine Flow Targets" {
            n99 = Unbundle By Name(w309) -> ("Pump State"=w312:bool, "Valve 1 State"=w311:bool)
            n100 = case "Pump On?" shown="True" w312 {
              tunnel: [w316 w320] -> w307
              tunnel: [w317 w319] -> w306
              tunnel: w311 -> [_ w323]
              frame False {
                w317 = 0.0  # Flow 2
                w316 = 0.0  # Flow 1
                # "If Pump is OFF, simulate no flow for either meter"
              }
              frame True {
                # "Simulated flow setpoint data"
                n101 = Select(t=9.0, s=w323, f=0.0) -> (s? t:f=w319:dbl)
                n102 = Subtract(x=20.0, y=w319) -> (x-y=w320:dbl)
              }
            }
            n103 = Bundle By Name(cluster=w309, "Flow 1 Target"=w307, "Flow 2 Target"=w306) -> (w308:T5)
            n104 = call <vilib>:"Add State(s) to Queue__jki_lib_state_machine.vi"("State(s) in (\"\")"=w315) -> ("States Out"=w314:string)  [unwired: 14 in]
          }
          frame "API: Determine Actual Flow" {
            # "asymptotically appraoch target value with each iteration"
            # "If target value for either is 0, don't add noise to that particular channel."
            # "Simulate flow rate data"
            n105 = Unbundle By Name(w347) -> ("Flow 1 Target"=w335:dbl, "Flow 1 Actual"=w336:dbl, "Flow 2 Target"=w324:dbl, "Flow 2 Actual"=w334:dbl)
            n106 = Equal To 0?(x=w335) -> (x = 0?=w328:bool)
            n107 = Equal To 0?(x=w324) -> (x = 0?=w332:bool)
            n108 = Random Number (0-1)() -> (number: 0 to 1=w329:dbl)
            n109 = Random Number (0-1)() -> (number: 0 to 1=w331:dbl)
            n110 = Select(t=0.0, s=w328, f=w329) -> (s? t:f=w326:dbl)
            n111 = Select(t=0.0, s=w332, f=w331) -> (s? t:f=w325:dbl)
            n112 = Subtract(x=w335, y=w336) -> (x-y=w345:dbl)
            n113 = Subtract(x=w324, y=w334) -> (x-y=w340:dbl)
            n114 = Divide(x=w345, y=4.0) -> (x/y=w343:dbl)
            n115 = Divide(x=w340, y=3.0) -> (x/y=w338:dbl)
            n116 = Add(x=w336, y=w343) -> (x+y=w342:dbl)
            n117 = Add(x=w334, y=w338) -> (x+y=w333:dbl)
            n118 = Add(x=w326, y=w342) -> (x+y=w341:dbl)
            n119 = Add(x=w333, y=w325) -> (x+y=w337:dbl)
            n120 = Bundle By Name(cluster=w347, "Flow 1 Actual"=w341, "Flow 2 Actual"=w337) -> (w346:T5)
            n121 = call <vilib>:"Add State(s) to Queue__jki_lib_state_machine.vi"("State(s) in (\"\")"=w351) -> ("States Out"=w350:string)  [unwired: 14 in]
          }
          frame "API: Update State" {
            n122 = Unbundle By Name(w357) -> ("Self Ref"=w356:refnum<class "SMO.Example.lvclass">, "Flow 1 Actual"=w353:dbl, "Flow 2 Actual"=w352:dbl)
            n123 = call "SMO.Example.SetData.vi"("error in (no error)"=w355, "Flow 2"=w352, "Flow 1"=w353, "SMO.Example"=w356) -> ("error out"=w354:errorcluster)  [unwired: 6 in, 1 out]
            n124 = call <vilib>:"Add State(s) to Queue__jki_lib_state_machine.vi"("State(s) in (\"\")"=w360) -> ("States Out"=w359:string)  [unwired: 14 in]
          }
        }
      }
    }
    frame Error {
    }
  }
  n125 = call-parent "Process.vi"("error in"=w8, "SMO"=w7) -> ("error out"=w5:errorcluster, "SMO out"=→"SMO.Example out":refnum<class "SMO.Example.lvclass">)  [unwired: 8 in]
  n126 = Merge Errors(w5, w4) -> (→"error out":errorcluster)
